vi "task.vi"   [LabVIEW 2016, in "斯坦道原位多参数.lvlib"]
types:
  T1 = typedef "斯坦道原位多参数.lvlib/水样测试启动自定义输入参数.ctl" = cluster{"测量模式":string, "数据类型":string}
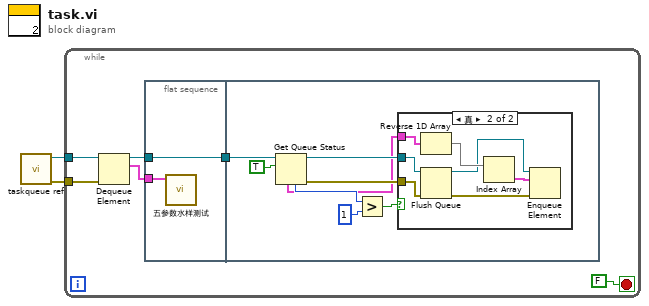
[diagram p0: block diagram]
diagram:
  n1 = call "taskqueue ref.vi"() -> ("错误输出"=w1:errorcluster, "队列输出"=w2:refnum<queue>)  [unwired: 10 in]
  n2 = while {
    tunnel: w2 -> [w8]
    tunnel: w1 -> [w7]
    stop <- FALSE stop-if-true
    n3 = Dequeue Element(queue=w8, error in (no error)=w7) -> (queue out=w6:refnum<queue>, element=w5:T1)  [unwired: 1 in, 2 out]
    n4 = flat-sequence {
      tunnel: w6 -> [w9]
      tunnel: w5 -> [w10]
      tunnel: [w9] -> w4
      tunnel: w4 -> [w18]
      frame #0 {
        n5 = call "五参数水样测试.vi"("启动参数"=w10) -> ()  [unwired: 11 in]
      }
      frame #1 {
        n6 = Get Queue Status(queue=w18, return elements? (F)=TRUE ("返回元素？(F)")) -> (queue out=w13:refnum<queue>, error out=w12:errorcluster, # elements in queue=w16:i32, elements=w11:T1[])  [unwired: 1 in, 4 out]
        n7 = Greater?(x=w16, y=1) -> (0:w14:bool)
        n8 = case shown="真" w14 {
          tunnel: w13 -> [_ w25]
          tunnel: w12 -> [_ w24]
          tunnel: w11 -> [_ w23]
          frame False {
          }
          frame True {
            n9 = Reverse 1D Array(array=w23) -> (reversed array=w22:T1[])
            n10 = Flush Queue(queue=w25, error in (no error)=w24) -> (queue out=w21:refnum<queue>, error out=w20:errorcluster)  [unwired: 1 out]
            n11 = Index Array(array=w22) -> (element=w19:T1)  [unwired: 1 in]
            n12 = Enqueue Element(queue=w21, element=w19, error in (no error)=w20) -> ()  [unwired: 1 in, 3 out]
          }
        }
      }
    }
  }
